vi "build.vi"() -> ()   [LabVIEW 2015]
uses:
  <userlib>/antonio-alexander/lv-build-interface/lv-build-interface.lvlib
panel:
  out "error":errorcluster
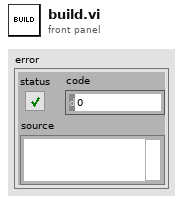
[diagram p1: front panel]
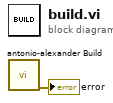
[diagram p0: block diagram]
diagram:
  n1 = call "antonio-alexander Build.vi"() -> ("error out"=→"error":errorcluster)  [unwired: 11 in]
